vi "CoMP-S Tune LCVR.vi"(6 "Beam":u16(ring)=1 items=["-1", "1"], 7 "Wavelength (nm)":dbl=1083.0 min=0.0 step=0.01 format="%.3f") -> (1 "Required LCVR Voltages":dbl[](array[numeric]) format="%.3f", 3 "Camera Choice":i32)   [LabVIEW 2014]
uses:
  CoMP-S Global.vi
panel:
  in  "SWIR Threshold Wavelength (900nm)":dbl=600.0
  out "Region Index":i32 caption="min index(es)"
  out "ld (nm)":dbl[](array[numeric]) format="%.5e"
  out "Order":dbl[](array[numeric])
  # "03-DEC-2013 = to be sure we're using Goodrich , treshold is set to 600!!!"
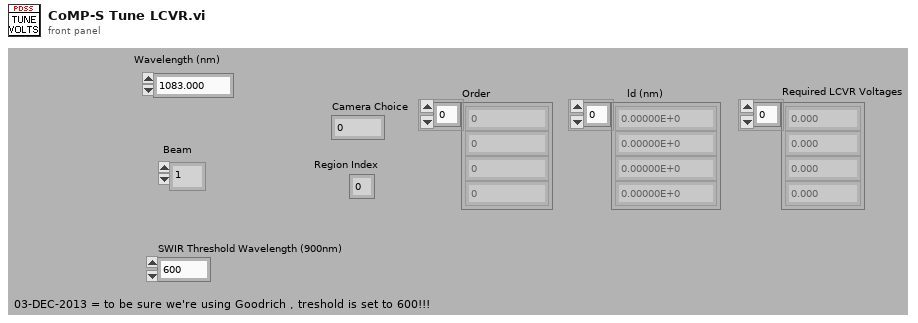
[diagram p1: front panel]
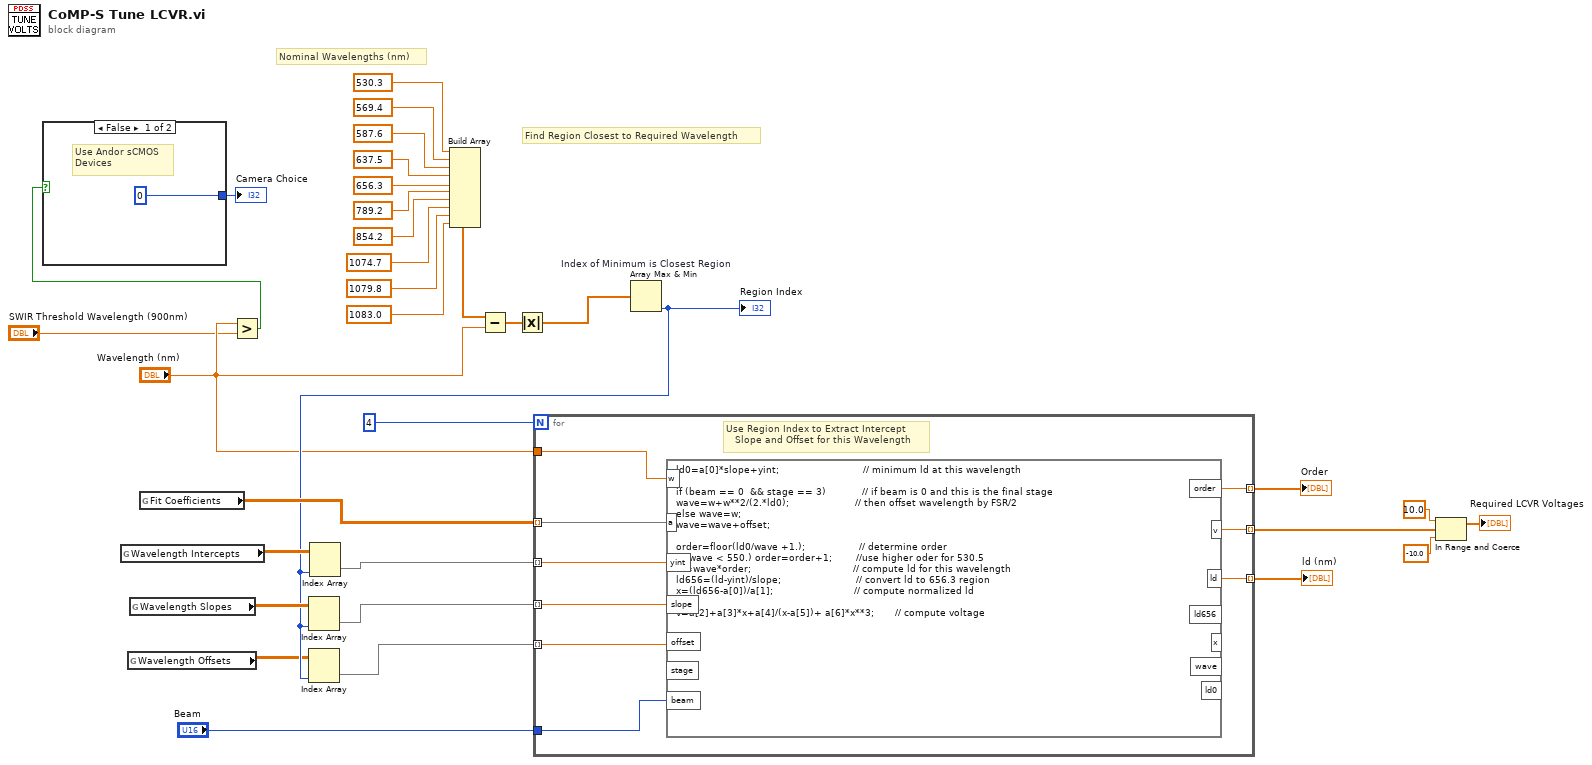
[diagram p0: block diagram]
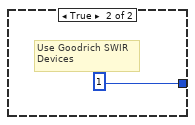
[diagram p2: hidden frame]
diagram:
  # "Find Region Closest to Required Wavelength"
  # "Nominal Wavelengths (nm)"
  n1 = global read "CoMP-S Global.vi" "Wavelength Intercepts"() -> (w16:dbl[][])
  n2 = global read "CoMP-S Global.vi" "Wavelength Offsets"() -> (w11:dbl[][])
  n3 = global read "CoMP-S Global.vi" "Wavelength Slopes"() -> (w15:dbl[][])
  n4 = global read "CoMP-S Global.vi" "Fit Coefficients"() -> (w17:dbl[][])
  n5 = Greater?(x="Wavelength (nm)", y="SWIR Threshold Wavelength (900nm)") -> (0:w6:bool)
  n6 = case shown="False" w6 {
    tunnel: [0 1] -> w5
    frame False {
      # "Use Andor sCMOS\nDevices"
    }
    frame True {
      # "Use Goodrich SWIR\nDevices"
    }
  }
  "Camera Choice" <- w5
  n7 = Build Array(530.3 ("element"), 569.4 ("element"), 587.6 ("element"), 637.5 ("element"), 656.3 ("element"), 789.2 ("element"), 854.2 ("element"), 1074.7 ("element"), 1079.8 ("element"), 1083.0 ("element")) -> (w30:dbl[])
  n8 = Subtract(x=w30, y="Wavelength (nm)") -> (x-y=w29:dbl[])
  n9 = Absolute Value(x=w29) -> (abs(x)=w18:dbl[])
  n10 = Array Max & Min "Index of Minimum is Closest Region"(array=w18) -> (min index (indices)=w12:i32)  [unwired: 3 out]
  "Region Index" <- w12
  n11 = Index Array(array=w15, index (col)=w12) -> (element=w13:dbl[])  [unwired: 1 in]
  n12 = Index Array(array=w11, index (col)=w12) -> (element=w10:dbl[])  [unwired: 1 in]
  n13 = Index Array(array=w16, index (col)=w12) -> (element=w14:dbl[])  [unwired: 1 in]
  n14 = for {
    N: 4 -> [_]
    tunnel: w17 -> [w45] mode=indexing
    tunnel: [w44] -> w1 mode=indexing
    tunnel: [w43] -> w32 mode=indexing
    tunnel: [w42] -> w33 mode=indexing
    tunnel: "Beam" -> [w40]
    tunnel: "Wavelength (nm)" -> [w39]
    tunnel: w14 -> [w37] mode=indexing
    tunnel: w13 -> [w38] mode=indexing
    tunnel: w10 -> [w36] mode=indexing
    i -> [w41]
    # "Use Region Index to Extract Intercept\n   Slope and Offset for this Wavelength"
    n15 = formula code="ld0=a[0]*slope+yint;                            // minimum ld at this wavelength\n\nif (beam == 0  && stage == 3)            // if beam is 0 and this is the final stage\nwave=w+w**2/(2.*ld0);                      // then offset wavelength by FSR/2\nelse wave=w;\nwave=wave+offset;\n\norder=floor(ld0/wave +1.);                  // determine order\nif (wave < 550.) order=order+1;        //use higher oder for 530.5\nld=wave*order;                                  // compute ld for this wavelength\nld656=(ld-yint)/slope;                         // convert ld to 656.3 region\nx=(ld656-a[0])/a[1];                           // compute normalized ld\n\nv=a[2]+a[3]*x+a[4]/(x-a[5])+ a[6]*x**3;       // compute voltage"("a"=w45, "w"=w39, "stage"=w41, "beam"=w40, "slope"=w38, "yint"=w37, "offset"=w36) -> ("order"=w42:dbl, "v"=w44:dbl, "ld"=w43:dbl)  [unwired: 4 out]
  }
  "Order" <- w33
  "ld (nm)" <- w32
  n16 = In Range and Coerce(upper limit=10.0, x=w1, lower limit=-10.0) -> (coerced(x)=→"Required LCVR Voltages":dbl[])  [unwired: 1 out]
